vi "Clear String.vi"(8 "Error In":errorcluster, 11 "String Ref":refnum<vi>) -> (0 "Error Out":errorcluster)   [LabVIEW 2022 SP3]
doc: "This VI clears the contents of a String object (control or indicator)."
panel:
  # "Development\nControls or indicators that are useful for development or testing, but which are not outputs of the VI."
  # "Input\nInputs to the VI"
  # "Output\nOutputs of the VI"
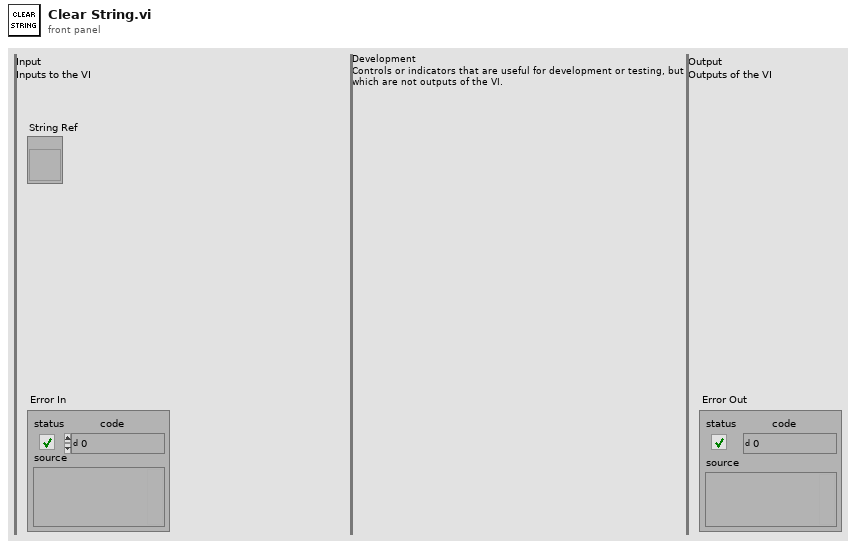
[diagram p1: front panel]
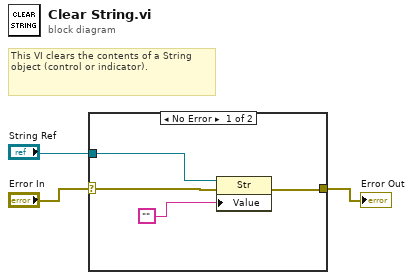
[diagram p0: block diagram]
diagram:
  # "This VI clears the contents of a String object (control or indicator)."
  n1 = case shown="No Error" "Error In" {
    selector: "Error In" -> [w6 w8]
    tunnel: [w5 w8] -> w2
    tunnel: "String Ref" -> [w4 _]
    frame No Error {
      n2 = property class="Str"(reference=w4, error in=w6, "Value"="") -> (error out=w5:errorcluster)  [unwired: 1 out]
    }
    frame Error {
    }
  }
  "Error Out" <- w2
